vi "CreateProjectsForEachLibrary.vi"() -> ()   [LabVIEW 2019, in "HawkeyeToolsMenu.lvlib"]
uses:
  HawkeyeToolsMenu.lvlib
  <userlib>/_OpenG.lib/file/file.llb/Valid Path - Traditional__ogtk.vi
  vi.lib/Hawkeye/Hawkeye.lvlib
panel:
  out "ExpectedDeps Files Created Created":path[](array[path])
  out "Projects Created":path[](array[path])
  out "error out":errorcluster
  in  "Build Specs Folder Path":path=path "C:/sw-deps-monitor/Source/BuildSpecs"
  in  "error in (no error)":errorcluster
  in  "Source Folder Path":path=path "C:/sw-deps-monitor/Source"
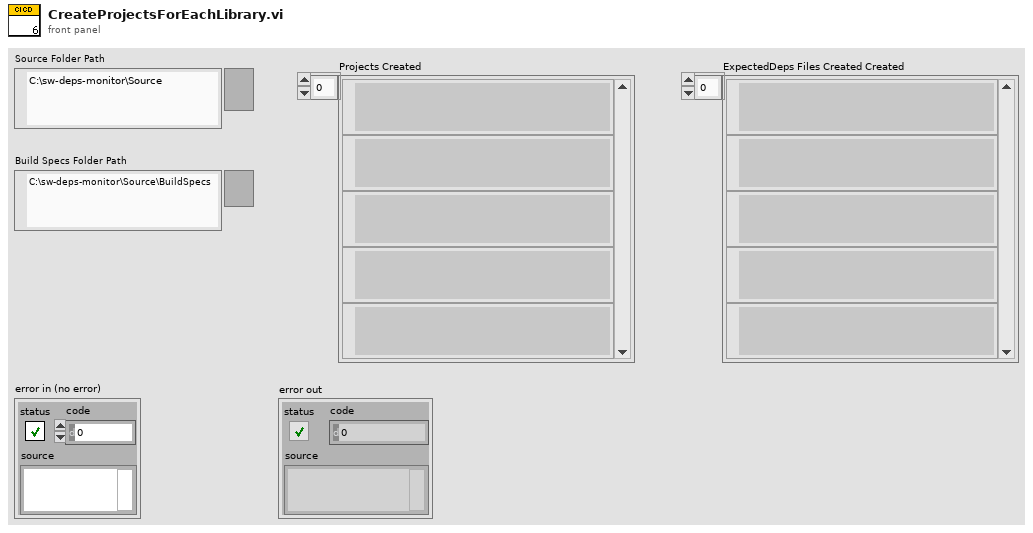
[diagram p1: front panel]
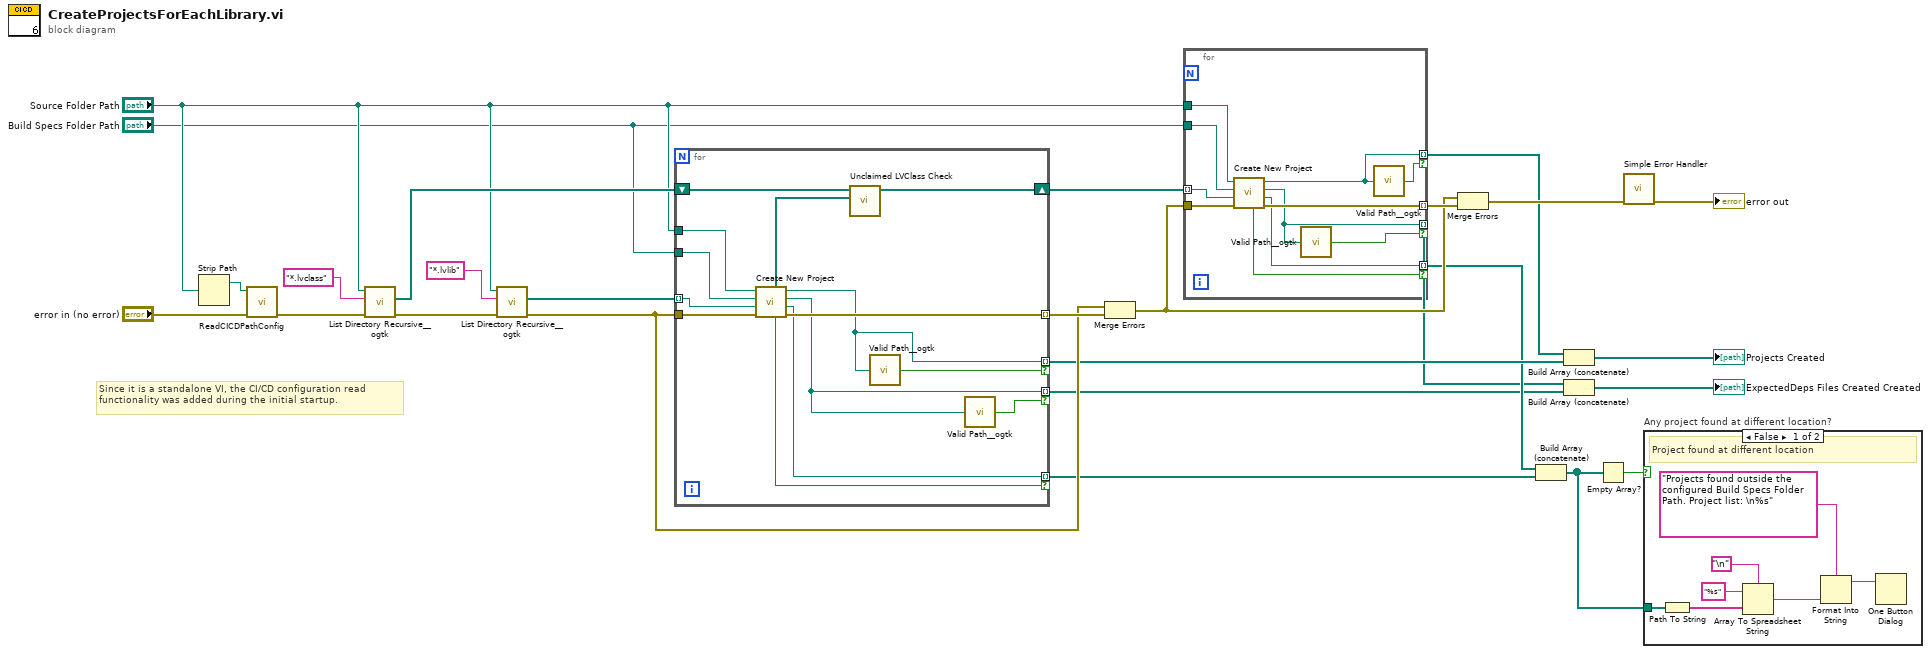
[diagram p0: block diagram]
diagram:
  # "Since it is a standalone VI, the CI/CD configuration read functionality was added during the initial startup."
  n1 = Strip Path(path="Source Folder Path") -> (stripped path=w20:path)  [unwired: 1 out]
  n2 = call "ReadCICDPathConfig.vi"("error in (no error)"="error in (no error)", "Workspace Path"=w20) -> ("error out"=w10:errorcluster)  [unwired: 8 in, 1 out]
  n3 = call <userlib>:"List Directory Recursive__ogtk.vi"("error in (no error)"=w10, "pattern"="*.lvclass", "Path"="Source Folder Path") -> ("error out"=w19:errorcluster, "file paths"=w17:path[])  [unwired: 5 in, 2 out]
  n4 = call <userlib>:"List Directory Recursive__ogtk.vi"("error in (no error)"=w19, "pattern"="*.lvlib", "Path"="Source Folder Path") -> ("error out"=w24:errorcluster, "file paths"=w26:path[])  [unwired: 5 in, 2 out]
  n5 = for {
    tunnel: w24 -> [w35]
    tunnel: w26 -> [w38] mode=indexing
    tunnel: "Build Specs Folder Path" -> [w39]
    tunnel: [w36] -> w25 mode=indexing
    tunnel: [w28] -> w23 mode=indexing if=w30
    tunnel: "Source Folder Path" -> [w37]
    tunnel: [w33] -> w21 mode=indexing if=w34
    shift-right: [w40] -> w16
    shift-left: w17 -> [w41]
    tunnel: [w32] -> w4 mode=indexing if=w31
    n6 = call "Create New Project.vi"("error in (no error)"=w35, "File Path to Append"=w38, "Build Specs Folder Path"=w39, "Source Folder Path"=w37) -> ("error out"=w36:errorcluster, "Project Mismatch Path"=w33:path, "ExpectedDeps Files Created"=w32:path, "Project Created"=w28:path, "Project Path Mismatch?"=w34:bool, "Owned Class[]"=w29:path[])  [unwired: 2 in]
    n7 = call "Unclaimed LVClass Check.vi"("Claimed Class"=w29, "Class Path List In"=w41) -> ("Class Path List Out"=w40:path[])  [unwired: 9 in]
    n8 = call-poly <userlib>:"Valid Path__ogtk.vi"("path"=w28) -> ("valid"=w30:bool)
    n9 = call-poly <userlib>:"Valid Path__ogtk.vi"("path"=w32) -> ("valid"=w31:bool)
  }
  n10 = Merge Errors(w24, w25) -> (w13:errorcluster)
  n11 = for {
    tunnel: "Source Folder Path" -> [w52]
    tunnel: "Build Specs Folder Path" -> [w51]
    tunnel: w16 -> [w50] mode=indexing
    tunnel: w13 -> [w49]
    tunnel: [w48] -> w15 mode=indexing
    tunnel: [w46] -> w8 mode=indexing if=w47
    tunnel: [w42] -> w7 mode=indexing if=w43
    tunnel: [w44] -> w3 mode=indexing if=w45
    n12 = call "Create New Project.vi"("error in (no error)"=w49, "File Path to Append"=w50, "Build Specs Folder Path"=w51, "Source Folder Path"=w52) -> ("error out"=w48:errorcluster, "Project Mismatch Path"=w46:path, "ExpectedDeps Files Created"=w44:path, "Project Created"=w42:path, "Project Path Mismatch?"=w47:bool)  [unwired: 2 in, 1 out]
    n13 = call-poly <userlib>:"Valid Path__ogtk.vi"("path"=w44) -> ("valid"=w45:bool)
    n14 = call-poly <userlib>:"Valid Path__ogtk.vi"("path"=w42) -> ("valid"=w43:bool)
  }
  n15 = Merge Errors(w13, w15) -> (w14:errorcluster)
  n16 = Build Array (concatenate)(w8, w21) -> (w6:path[])
  n17 = Build Array (concatenate)(w7, w23) -> (→"Projects Created":path[])
  n18 = Build Array (concatenate)(w3, w4) -> (→"ExpectedDeps Files Created Created":path[])
  n19 = Empty Array?(array=w6) -> (empty?=w22:bool)
  n20 = call <vilib>:"Simple Error Handler.vi"("error in (no error)"=w14) -> ("error out"=→"error out":errorcluster)  [unwired: 4 in, 4 out]
  n21 = case "Any project found at different location?" shown="False" w22 {
    tunnel: w6 -> [w59 _]
    frame False {
      # "Project found at different location"
      n22 = Path To String(path=w59) -> (string=w56:string[])
      n23 = Array To Spreadsheet String(delimiter (Tab)="\n", array=w56, 3:"%s" ("format string")) -> (spreadsheet string=w55:string)
      n24 = Format Into String(format string="Projects found outside the configured Build Specs Folder Path. Project list: \n%s", w55) -> (resulting string=w54:string)  [unwired: 2 in, 1 out]
      n25 = One Button Dialog(message=w54) -> ()  [unwired: 1 in, 1 out]
    }
    frame True {
    }
  }
